vi "UART 8N1 Wait Response.vi"(7 "Active Dut":T1, 8 "Response Size (char)":u32, 9 "Response Timeout (ms)":i32, 10 "Error In":errorcluster, 11 "FPGA VI Reference In":refnum<k20>) -> (0 "Received Text":string, 1 "Timeout Flag":bool, 2 "Error Out":errorcluster, 3 "FPGA VI Reference Out":refnum<k20>, 5 "Elements Remaining":u32)   [LabVIEW 2018]
uses:
  Resources_Test/UART/ControlTestSlot.ctl
  <vilib>/Utility/error.llb/Error Cluster From Error Code.vi
  <vilib>/rvi/errors/niLvFpgaAdjustHostInterfaceError.vi
  <vilib>/rvi/interface/nirviMethod/nirviMethod.xnode
  Program Files (x86)/National Instruments/LabVIEW 2018/instr.lib/niVST/FPGA/Templates/FPGA Bitfiles/niVSTFPGA_UART.lvbitx
  <vilib>/rvi/errors/niLvFpgaMergeErrorWithErrorCode.vi
  <vilib>/FPGAPlugInAG/PXIe-5840/niLvFpga_ReadFifo_PXIe-5840.vi
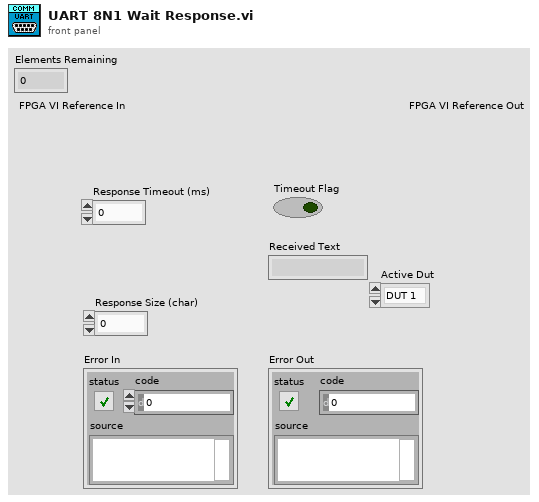
[diagram p1: front panel]
types:
  T1 = typedef "ControlTestSlot.ctl" = enum16{"DUT 1", "DUT 2"}
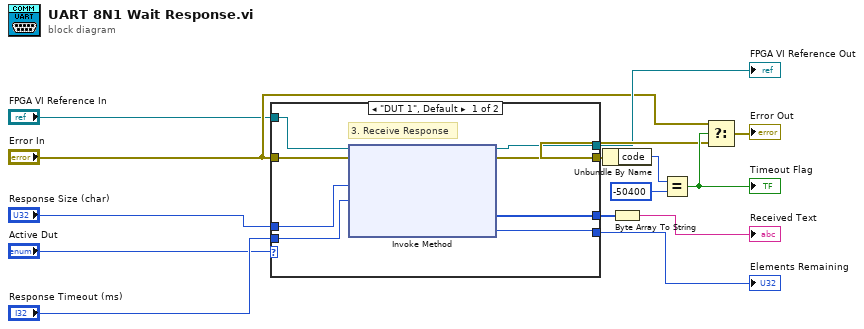
[diagram p0: block diagram]
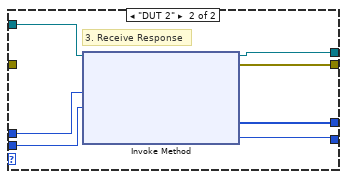
[diagram p2: hidden frame]
diagram:
  n1 = case shown="\"DUT 1\", Default" "Active Dut" {
    tunnel: "Error In" -> [w16 _]
    tunnel: [w22 w29] -> w5
    tunnel: [w21 w28] -> w6
    tunnel: "Response Size (char)" -> [w20 w27]
    tunnel: "Response Timeout (ms)" -> [w19 w26]
    tunnel: [w18 w25] -> w7
    tunnel: [w17 w24] -> w4
    tunnel: "FPGA VI Reference In" -> [w15 w23]
    frame "DUT 1", Default {
      # "3. Receive Response"
      n2 = xnode "Invoke Method"("FPGA VI Reference In"=w15, "error in"=w16, "Number of Elements"=w20, "Timeout (ms)"=w19) -> ("FPGA VI Reference Out"=w22:refnum<k20>, "error out"=w21:errorcluster, "Data"=w18:u32[], "Elements Remaining"=w17:u32)
    }
    frame "DUT 2" {
      # "3. Receive Response"
      n3 = xnode "Invoke Method"("FPGA VI Reference In"=w23, "Number of Elements"=w27, "Timeout (ms)"=w26) -> ("FPGA VI Reference Out"=w29:refnum<k20>, "error out"=w28:errorcluster, "Data"=w25:u32[], "Elements Remaining"=w24:u32)  [unwired: 1 in]
    }
  }
  "FPGA VI Reference Out" <- w5
  "Elements Remaining" <- w4
  n4 = Unbundle By Name(w6) -> ("code"=w12:i32)
  n5 = Byte Array To String(unsigned byte array=w7) -> (string=→"Received Text":string)
  n6 = Equal?(x=w12, y=-50400) -> (x = y?=w10:bool)
  "Timeout Flag" <- w10
  n7 = Select(t="Error In", s=w10, f=w6) -> (s? t:f=→"Error Out":errorcluster)
